vi "test_Format String to Numeric_U32 value flattened.vi"(8 "error in (no error)":errorcluster, 11 "TestCase in":refnum<class "Instrument Addon Unit Tests.lvclass">) -> (0 "error out":errorcluster, 3 "TestCase out":refnum<class "Instrument Addon Unit Tests.lvclass">)   [LabVIEW 2019, in "Instrument Addon Unit Tests.lvclass"]
uses:
  Instrument Addon Unit Tests.lvclass
  Addon/Addon Shared/Types/Endian.ctl
  Addon/Addon Shared/Types/Data Channel Type.ctl
  Addon/Addon Shared/Types/Type Cast Type.ctl
  <vilib>/addons/_JKI Toolkits/VI Tester/TestCase.llb/TestCase.lvclass
  Addon/Addon Engine/Instrument Addon Engine.lvlib
  Addon/Addon Shared/Instrument Addon Shared.lvlib
  C:/Program Files (x86)/National Instruments/LabVIEW 2019/vi.lib/addons/_JKI Toolkits/VI Tester/TestCase.llb/TestCase.lvclass
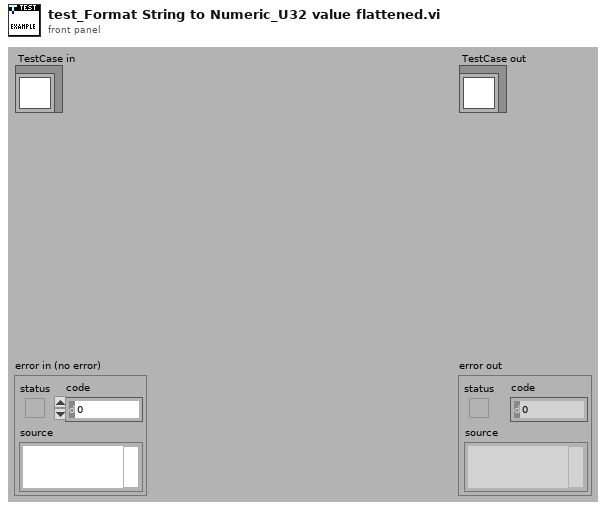
[diagram p1: front panel]
types:
  T1 = typedef "Instrument Addon Shared.lvlib/Type Cast Type.ctl" = enum16{"DBL", "SGL", "U64", "U32", "U16", "U8", "I64", "I32", "I16", "I8"}
  T2 = typedef "Instrument Addon Shared.lvlib/Data Channel Type.ctl" = enum16{"Format", "Comparison", "Type Cast", "Enumerated List"}
  T3 = typedef "Instrument Addon Shared.lvlib/Endian.ctl" = enum16{"Native", "Little", "Big"}
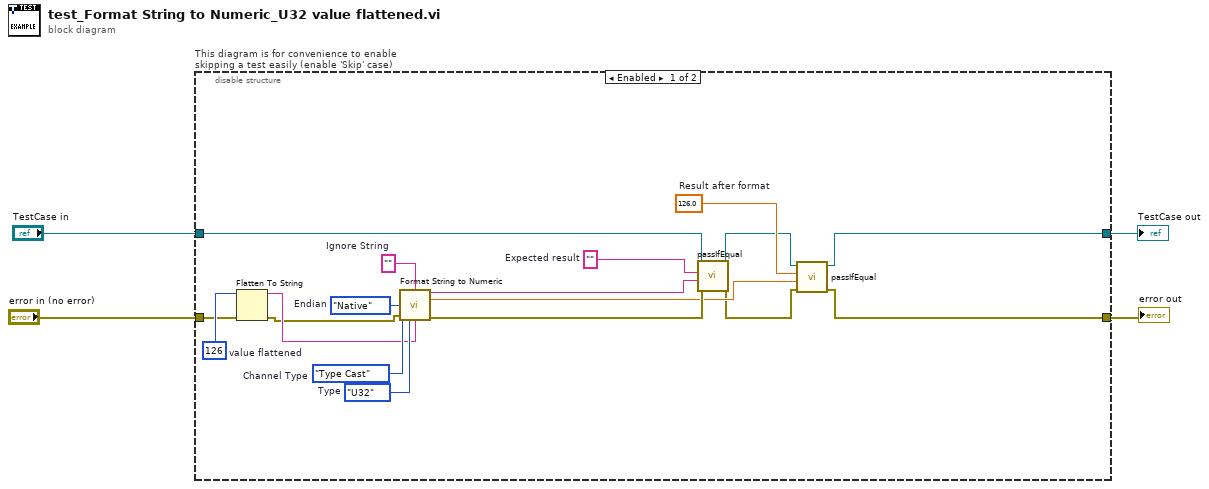
[diagram p0: block diagram]
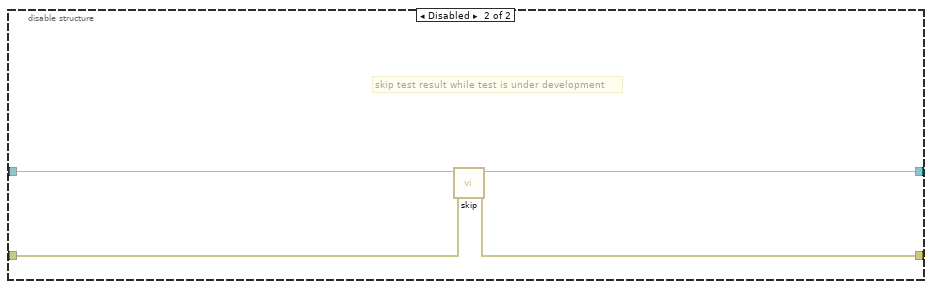
[diagram p2: hidden frame]
diagram:
  n1 = disable-structure "This diagram is for convenience to enable skipping a test easily (enable 'Skip' case)" shown="Enabled" {
    disable-tunnel: "TestCase in" -> [w22 w26]
    disable-tunnel: [w11 w24] -> w1
    disable-tunnel: [w13 w25] -> w3
    disable-tunnel: "error in (no error)" -> [w6 w23]
    frame Enabled {
      w8 = u32 126  # value flattened
      w9 = ""  # Ignore String
      w10 = Type_Cast_Type."U32"  # Type
      w15 = 126.0  # Result after format
      w17 = Data_Channel_Type."Type Cast"  # Channel Type
      w18 = ""  # Expected result
      w20 = Endian."Native"  # Endian
      n2 = Flatten To String(anything=w8, error in (no error)=w6) -> (data string=w7:string, error out=w5:errorcluster)  [unwired: 2 in, 1 out]
      n3 = call "Format String to Numeric.vi"("Ignore String"=w9, "Endian"=w20, "Channel Type"=w17, "error in (no error)"=w5, "Type"=w10, "Response"=w7) -> ("remaining string"=w19:string, "Value"=w16:dbl, "error out"=w21:errorcluster)  [unwired: 7 in]
      n4 = call-dynamic "passIfEqual.vi"("error in (no error)"=w21, "y"=w19, "x"=w18, "TestCase in"=w22) -> ("error out"=w14:errorcluster, "TestCase out"=w12:refnum<class "Instrument Addon Unit Tests.lvclass">)  [unwired: 6 in]
      n5 = call-dynamic "passIfEqual.vi"("error in (no error)"=w14, "y"=w16, "x"=w15, "TestCase in"=w12) -> ("error out"=w13:errorcluster, "TestCase out"=w11:refnum<class "Instrument Addon Unit Tests.lvclass">)  [unwired: 6 in]
    }
    frame Disabled {
      # "skip test result while test is under development"
      n6 = call <vilib>:"skip.vi"("error in (no error)"=w23, "TestCase in"=w26) -> ("error out"=w25:errorcluster, "TestCase out"=w24:refnum<class "Instrument Addon Unit Tests.lvclass">)  [unwired: 8 in]
    }
  }
  "error out" <- w3
  "TestCase out" <- w1
